vi "vaisalaReadExtractSerial.vi"(8 "error in (no error)":errorcluster, 11 "VISA Refnum in":refnum<visa-resource-name>) -> (0 "error out":errorcluster, 1 "RH (%)":dbl, 2 "T (C)":dbl, 3 "VISA Refnum out":refnum<visa-resource-name>, 4 "Dp (C)":dbl)   [LabVIEW 2011]
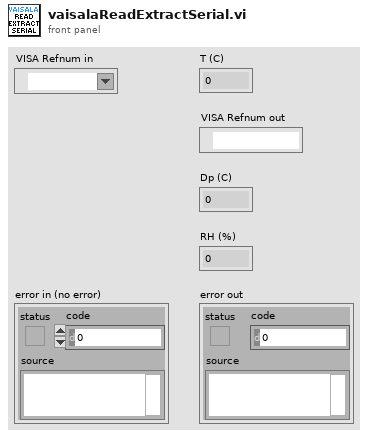
[diagram p1: front panel]
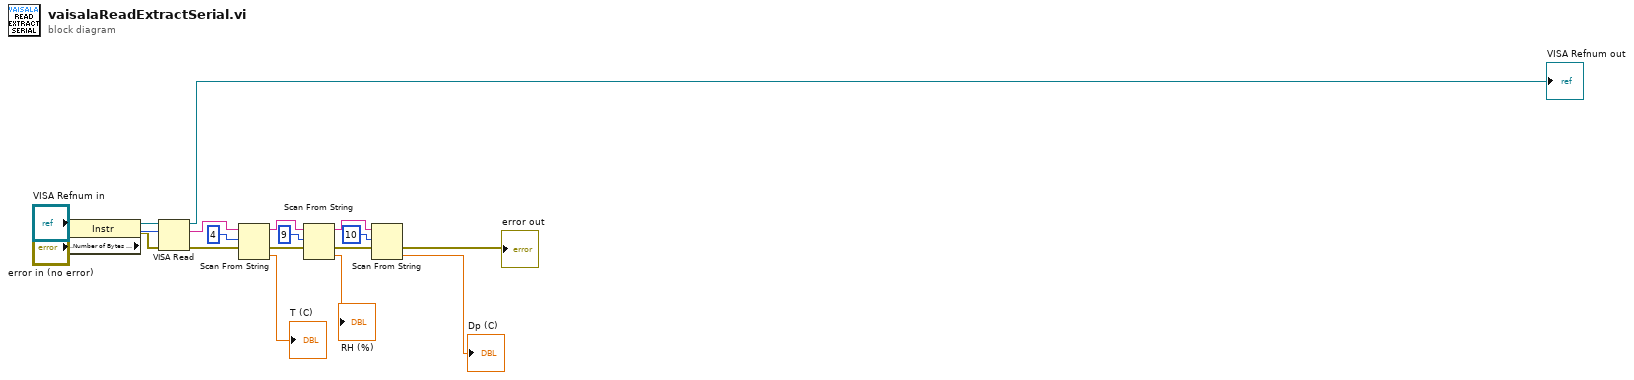
[diagram p0: block diagram]
diagram:
  n1 = property class="Instr"(reference="VISA Refnum in", error in="error in (no error)") -> (reference out=w4:refnum<visa-resource-name>, error out=w5:errorcluster, "Serial Settings:Number of Bytes at Serial Port"=w6:u32)
  n2 = VISA Read(VISA resource name=w4, byte count=w6, error in (no error)=w5) -> (VISA resource name out=→"VISA Refnum out":refnum<visa-resource-name>, read buffer=w15:string, error out=w7:errorcluster)  [unwired: 1 out]
  n3 = Scan From String(input string=w15, initial scan location=u32 4, error in=w7) -> (remaining string=w11:string, error out=w9:errorcluster, output 1=→"T (C)":dbl)  [unwired: 2 in, 1 out]
  n4 = Scan From String(input string=w11, initial scan location=u32 9, error in=w9) -> (remaining string=w13:string, error out=w10:errorcluster, output 1=→"RH (%)":dbl)  [unwired: 2 in, 1 out]
  n5 = Scan From String(input string=w13, initial scan location=u32 10, error in=w10) -> (error out=→"error out":errorcluster, output 1=→"Dp (C)":dbl)  [unwired: 2 in, 2 out]
